vi "מסך ניהול הייצור 1 8.11.vi"() -> ()   [LabVIEW 2013]
uses:
  <vilib>/Utility/file.llb/Read From Spreadsheet File (string).vi
panel:
  out ".not. (x .or. y)?":bool
  in  "hlpe arry to odrs 3":string[](array[string])
  out "current time":timestamp
  out "size(s)":i32[](array[numeric])
  out "index":i32[](array[numeric])
  out "element":string
  out "row":i32
  in  "cancel":bool
  in  "Go to production":bool
  in  "Order num for proudction":string(combo)
  out "Order List":string[][](array[string])
  # "Fider"
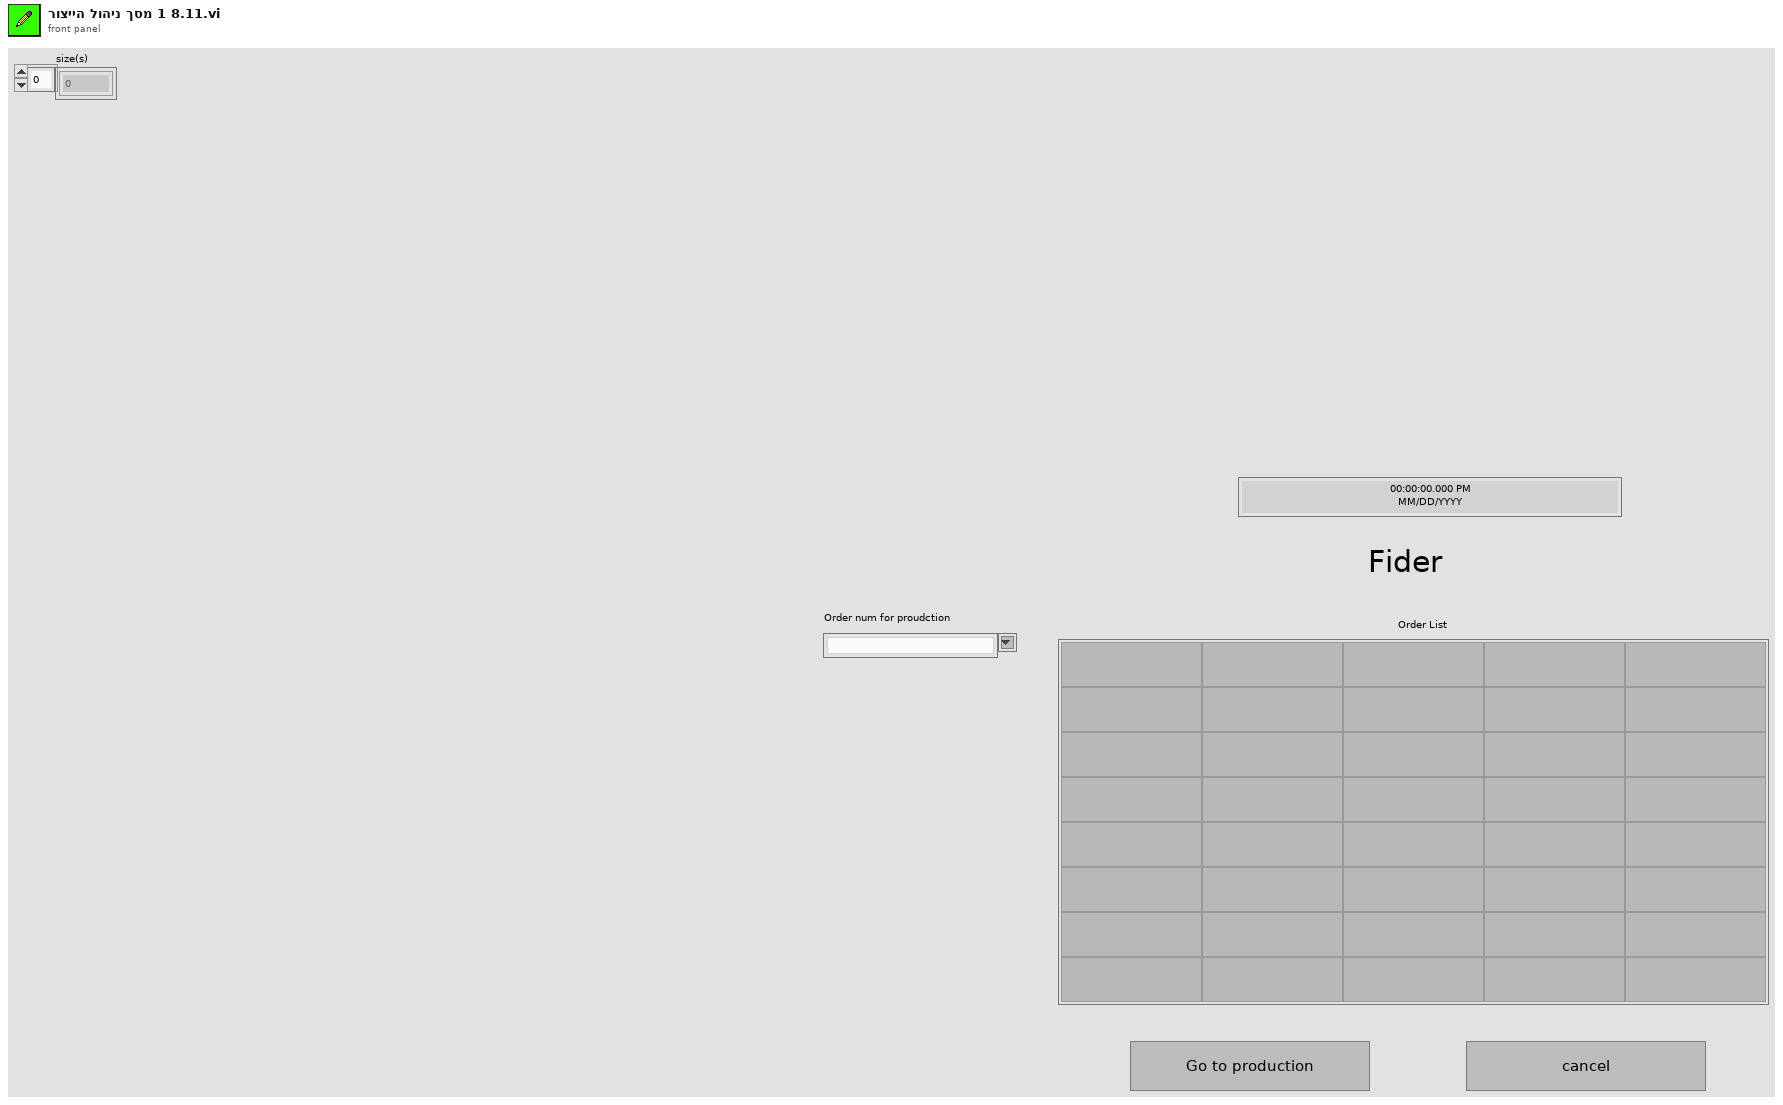
[diagram p1: front panel]
types:
  T1 = enum8{"Enabled", "Disabled", "Disabled and Grayed Out"}
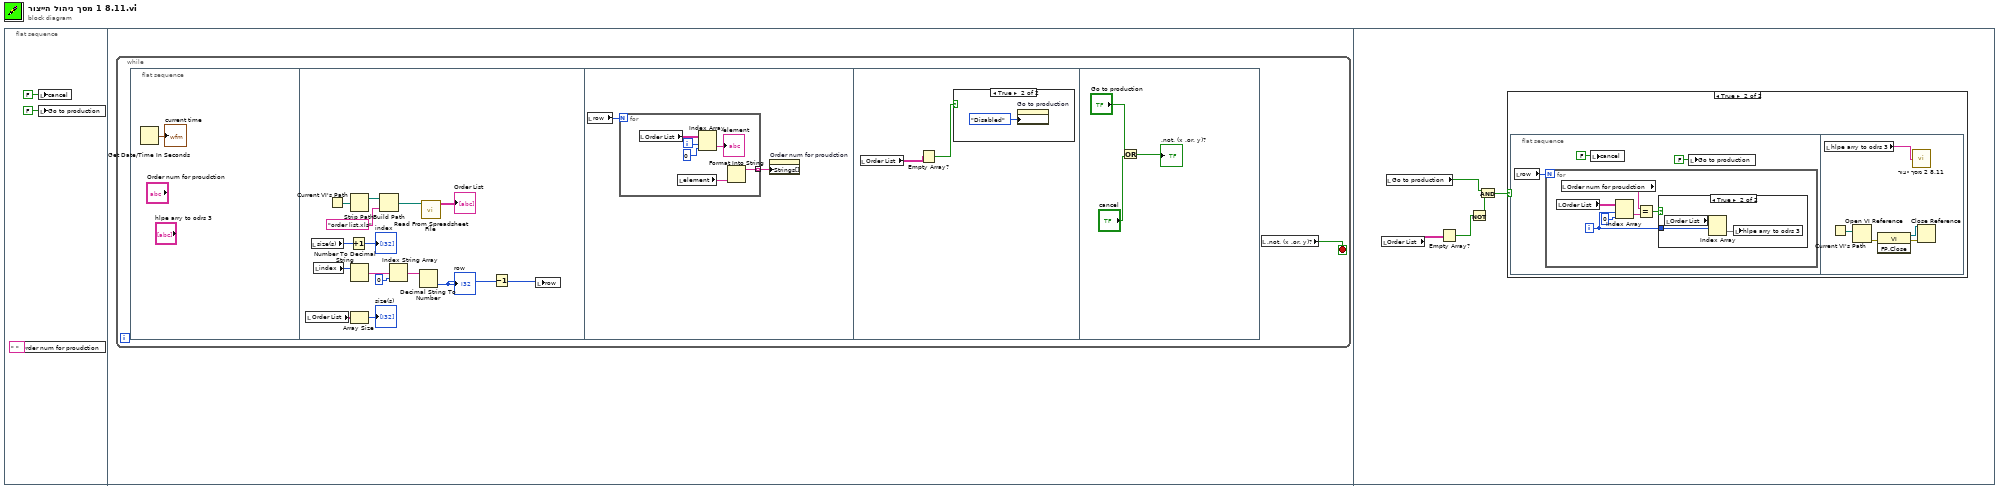
[diagram p0: block diagram]
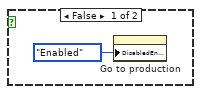
[diagram p2: hidden frame]
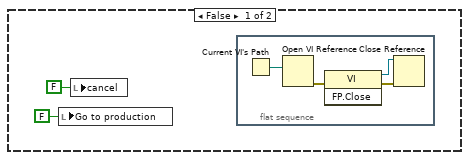
[diagram p3: hidden frame]
diagram:
  n1 = flat-sequence {
    frame #0 {
      n2 = local write "Order num for proudction"(" " ("Order num for proudction")) -> ()
      n3 = local write "cancel"(FALSE ("cancel")) -> ()
      n4 = local write "Go to production"(FALSE ("Go to production")) -> ()
    }
    frame #1 {
      n5 = while {
        stop <- w4 stop-if-true
        n6 = flat-sequence {
          frame #0 {
            n7 = Get Date/Time In Seconds() -> (seconds since 1Jan1904=→"current time":timestamp)
          }
          frame #1 {
            n8 = local read "Order List"() -> (w10:string[][])
            n9 = local read "size(s)"() -> (w12:i32[])
            n10 = local read "index"() -> (w16:i32[])
            n11 = Current VI's Path() -> (path=w18:path)
            n12 = Increment(x=w12) -> (x+1=→"index":i32[])
            n13 = Strip Path(path=w18) -> (stripped path=w19:path)  [unwired: 1 out]
            n14 = Number To Decimal String(number=w16) -> (decimal integer string=w15:string[])  [unwired: 1 in]
            n15 = Array Size(array=w10) -> (size(s)=→"size(s)":i32[])
            n16 = Build Path(base path=w19, name or relative path="order list.xls") -> (appended path=w20:path)
            n17 = Index String Array(1:0 ("index"), 2:w15) -> (0:w13:string)  [unwired: 1 in]
            n18 = Decimal String To Number(string=w13) -> (number=w7:i32)  [unwired: 2 in, 1 out]
            "row" <- w7
            n19 = call-poly <vilib>:"Read From Spreadsheet File.vi"("file path (dialog if empty)"=w20) -> ("all rows"=→"Order List":string[][])  [unwired: 6 in, 4 out]
            n20 = Decrement(x=w7) -> (x-1=w6:i32)
            n21 = local write "row"(w6) -> ()
          }
          frame #2 {
            n22 = local read "row"() -> (w21:i32)
            n23 = for {
              N: w21 -> [_]
              tunnel: [w28] -> w22 mode=indexing
              i -> [w27]
              n24 = local read "Order List"() -> (w24:string[][])
              n25 = local read "element"() -> (w25:string)
              n26 = Index Array(array=w24, index (row)=w27, index (col)=0 ("disabled index (col)")) -> (element=→"element":string)
              n27 = Format Into String(w25) -> (resulting string=w28:string)  [unwired: 3 in, 1 out]
            }
            n28 = property on="Order num for proudction" class="CmbBox"("Strings[]"=w22) -> ()  [unwired: 2 in, 2 out]
          }
          frame #3 {
            n29 = local read "Order List"() -> (w30:string[][])
            n30 = Empty Array?(array=w30) -> (empty?=w29:bool)
            n31 = case shown="True" w29 {
              frame False {
                n32 = property on="Go to production" class="Bool (strict)"("DisabledEnum"=T1."Enabled" ("Disabled")) -> ()  [unwired: 2 in, 2 out]
              }
              frame True {
                n33 = property on="Go to production" class="Bool (strict)"("DisabledEnum"=T1."Disabled" ("Disabled")) -> ()  [unwired: 2 in, 2 out]
              }
            }
          }
          frame #4 {
            n34 = Or(x="Go to production", y="cancel") -> (x .or. y?=→".not. (x .or. y)?":bool)
          }
        }
        n35 = local read ".not. (x .or. y)?"() -> (w4:bool)
      }
    }
    frame #2 {
      n36 = local read "Order List"() -> (w36:string[][])
      n37 = local read "Go to production"() -> (w40:bool)
      n38 = Empty Array?(array=w36) -> (empty?=w37:bool)
      n39 = Not(x=w37) -> (.not. x?=w38:bool)
      n40 = And(x=w40, y=w38) -> (x .and. y?=w39:bool)
      n41 = case shown="True" w39 {
        frame False {
          n42 = local write "Go to production"(FALSE ("Go to production")) -> ()
          n43 = local write "cancel"(FALSE ("cancel")) -> ()
          n44 = flat-sequence {
            frame #0 {
              n45 = Current VI's Path() -> (path=w46:path)
              n46 = Open VI Reference(vi path=w46) -> (error out=w45:errorcluster)  [unwired: 5 in, 1 out]
              n47 = invoke class="VI" method="FP.Close"(error in=w45) -> (reference out=w43:refnum<vi>, error out=w44:errorcluster)  [unwired: 2 in, 1 out]
              n48 = Close Reference(reference=w43, error in (no error)=w44) -> ()  [unwired: 1 out]
            }
          }
        }
        frame True {
          n49 = flat-sequence {
            frame #0 {
              n50 = local read "row"() -> (w49:i32)
              n51 = for {
                N: w49 -> [_]
                i -> [w50]
                n52 = local read "Order List"() -> (w54:string[][])
                n53 = local read "Order num for proudction"() -> (w55:string)
                n54 = Index Array(array=w54, index (row)=w50, index (col)=0 ("disabled index (col)")) -> (element=w52:string)
                n55 = Equal?(x=w55, y=w52) -> (x = y?=w51:bool)
                n56 = case shown="True" w51 {
                  tunnel: w50 -> [_ w57]
                  frame False {
                  }
                  frame True {
                    n57 = local read "Order List"() -> (w58:string[][])
                    n58 = Index Array(array=w58, index (row)=w57) -> (element=w56:string[])  [unwired: 1 in]
                    n59 = local write "hlpe arry to odrs 3"(w56) -> ()
                  }
                }
              }
              n60 = local write "cancel"(FALSE ("cancel")) -> ()
              n61 = local write "Go to production"(FALSE ("Go to production")) -> ()
            }
            frame #1 {
              n62 = local read "hlpe arry to odrs 3"() -> (w63:string[])
              n63 = Current VI's Path() -> (path=w62:path)
              n64 = Open VI Reference(vi path=w62) -> (error out=w61:errorcluster)  [unwired: 5 in, 1 out]
              n65 = invoke class="VI" method="FP.Close"(error in=w61) -> (reference out=w59:refnum<vi>, error out=w60:errorcluster)  [unwired: 2 in, 1 out]
              n66 = call "מסך ייצור 2 8.11.vi"("Order"=w63) -> ()  [unwired: 1 in]
              n67 = Close Reference(reference=w59, error in (no error)=w60) -> ()  [unwired: 1 out]
            }
          }
        }
      }
    }
  }
